vi "Main FPGA 8-axis.vi"() -> ()   [LabVIEW 2015]
uses:
  <vilib>/Motion/MotorControl/_s/nism.interpretControlRegister.stateTransition.ctl
  <vilib>/Platform/TimedLoop/XDataNode/timing_clust.ctl
  <vilib>/Platform/TimedLoop/XDataNode/nitl_modes.ctl
  <vilib>/Platform/TimedLoop/XDataNode/wakeup.ctl
  <vilib>/rvi/Emulation/niFpgaGetClockAttributes.vi
  <vilib>/rvi/Emulation/niFpgaSctlEmulationGetInTimedLoop.vi
  <vilib>/rvi/Emulation/niFpgaEmulationReportErrorSimple.vi
  Global FPGA 8-axis.vi
  <vilib>/Motion/MotorControl/_s/nism.interpretControlRegister.indexed.vi
  <vilib>/rvi/Emulation/niFpgaProcessEmulError.vi
  <vilib>/Motion/MotorControl/_s/nism.mdo.read.positionLoopSyncData.vi
  <vilib>/Motion/MotorControl/_s/nism.mdo.read.splineData.vi
  <vilib>/Motion/MotorControl/_s/nism.generateStatusRegister.indexed.vi
  <vilib>/rvi/eio/common/nirviEmuTemplateMethod_errors.vi
  <vilib>/rvi/Emulation/niFpgaCriticalErrorInLSC.vi
  <vilib>/Motion/MotorControl/_s/nism.splineInterpolation.fxp.3.index.vi
  <vilib>/Motion/MotorControl/_s/nism.mdo.handler.indexed.vi
  <vilib>/Motion/SoftMotion/Synchronization/nism.rioScan.generateSyncScan.vi
  <vilib>/eio/EIONode/EIONode.xnode
  <vilib>/Platform/TimedLoop/XDataNode/XDataNode.xnode
  <vilib>/Motion/MotorControl/NI_SoftMotion_MotorControlIP.lvlib
  <vilib>/Platform/TimedLoop/XDataNode/XDNodeRunTimeDep.lvlib
  <vilib>/Motion/SoftMotion/Synchronization/NI_SoftMotion_Synchronization.lvlib
panel:
  out "Interpolated Positions":fxp<+/-,64,32>[](array[numeric])
  out "Drive Enable":bool[](array[boolean])
  in  "Enable value":bool
  in  "Drive Enable override?":bool
  out "State":T1=enum."Start --> Initializing" caption="state transition"
  in  "Sync Value":bool
  in  "Sync Enable override?":bool
  in  "Invert direction?":bool
  out "Sync is Fault":bool
  out "Sync is Locked":bool
  in  "minimum pulse":u16=40
  # "Synchronization Loop"
  # "Control Status Loop"
  # "Notes: \n1. This VI provides the communication interface between the NI SoftMotion Engine and the LabVIEW FPGA Module. You must compile this VI for a specific FPGA target before use. After compiling, run the VI before running any of the Express VI examples. For information on moving this example to another FPGA target, refer to ni.com/info and enter info code fpgaex.\n\n2. Only use the Reset Axis button if you are unable to communicate with the axis by any other means. This button resets the device state machine and other VIs to a known state. After resetting the axis, switch the NI Scan Engine from Active Mode to Configuration Mode, then back to Active Mode, before attempting to enable the axis."
  # "(These two buttons \nare for testing\npurposes.)"
  # "(These two buttons \nare for testing\npurposes.)"
  # "Step/Direction Loop"
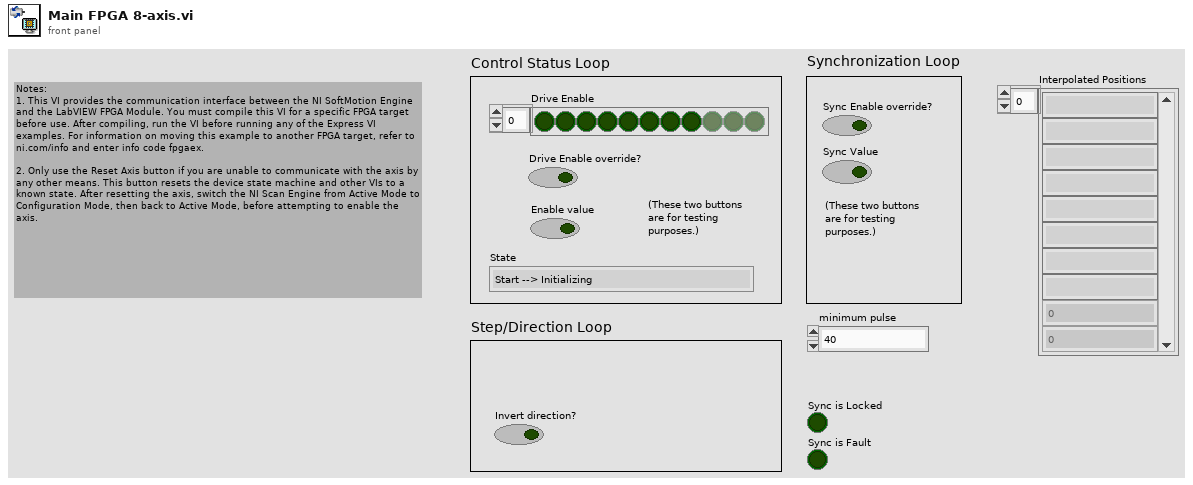
[diagram p1: front panel]
types:
  T1 = typedef "NI_SoftMotion_MotorControlIP.lvlib/nism.interpretControlRegister.stateTransition.ctl" = enum8{"Invalid", "Start --> Initializing", "Initializing --> Disabled", "Disabled --> Ready To Switch On", "Ready To Switch On --> Switched On", "Ready To Switch On --> Disable", "Switched On --> Operation Enable", "Switched On --> Ready To Switch On", "Switched On --> Disabled", "Operation Enable --> Switched On", "Operation Enable --> Ready To Switch On", "Operation Enable --> Disabled", "Fault --> Disabled", "Any --> Fault", "None"}
  T2 = typedef "NI_SoftMotion_MotorControlIP.lvlib/nism.mdo.splineData.ctl" = cluster{"spline type":T3, "traj per/spline per":u16, "spline per/traj per":fxp<+,32,0>}
  T3 = typedef "NI_SoftMotion_MotorControlIP.lvlib/nism.splineInterpolation.type.ctl" = u16
  T4 = typedef "NI_SoftMotion_Synchronization.lvlib/nism.softmotionScan.timerConfig.ctl" = cluster{"target period (clocks)":u16, "host period / target period":u16}
  T5 = typedef "NI_SoftMotion_Synchronization.lvlib/nism.softmotionScan.timerControl.ctl" = cluster{"sm scan":bool, "sm scan count":u32, "sm scan enabled":bool}
  T6 = typedef "XDNodeRunTimeDep.lvlib/timing_clust.ctl" = cluster{"Expected End [f-1]":u64, "Actual End [f-1]":u64, "Finished Late? [f-1]":bool, "Expected End [i-1]":u64, "Actual End [i-1]":u64, "Finished Late? [i-1]":bool, "Expected Start [i]":u64, "Actual Start [i]":u64, "Expected Start [f]":u64, "Actual Start [f]":u64, "Source Name":string, "Structure Name":string, "Period":i64, "Deadline":i64, "Offset":i64, "Start":i64, "Priority":i32, "Timeout":i32, "Mode":T7, "Wakeup Reason":T8, "Error":errorcluster, "Source Type":string, "Secondary Source Type":string, "Global End Time":u64, "Global Start Time":u64, "Frame Duration":u64, "Iteration Duration":u64, "Assigned CPU":i32, "I/O Scan Engine Mode":u32}
  T7 = typedef "XDNodeRunTimeDep.lvlib/nitl_modes.ctl" = enum32{"No Change", "Process missed periods, maintain original phase", "Discard missed periods, maintain original phase", "Process missed periods, ignore original phase", "Discard missed periods, ignore original phase"}
  T8 = typedef "XDNodeRunTimeDep.lvlib/wakeup.ctl" = enum32{"Normal", "Aborted", "Asynchronous wakeup", "Timing source error", "Timed loop error", "Timeout"}
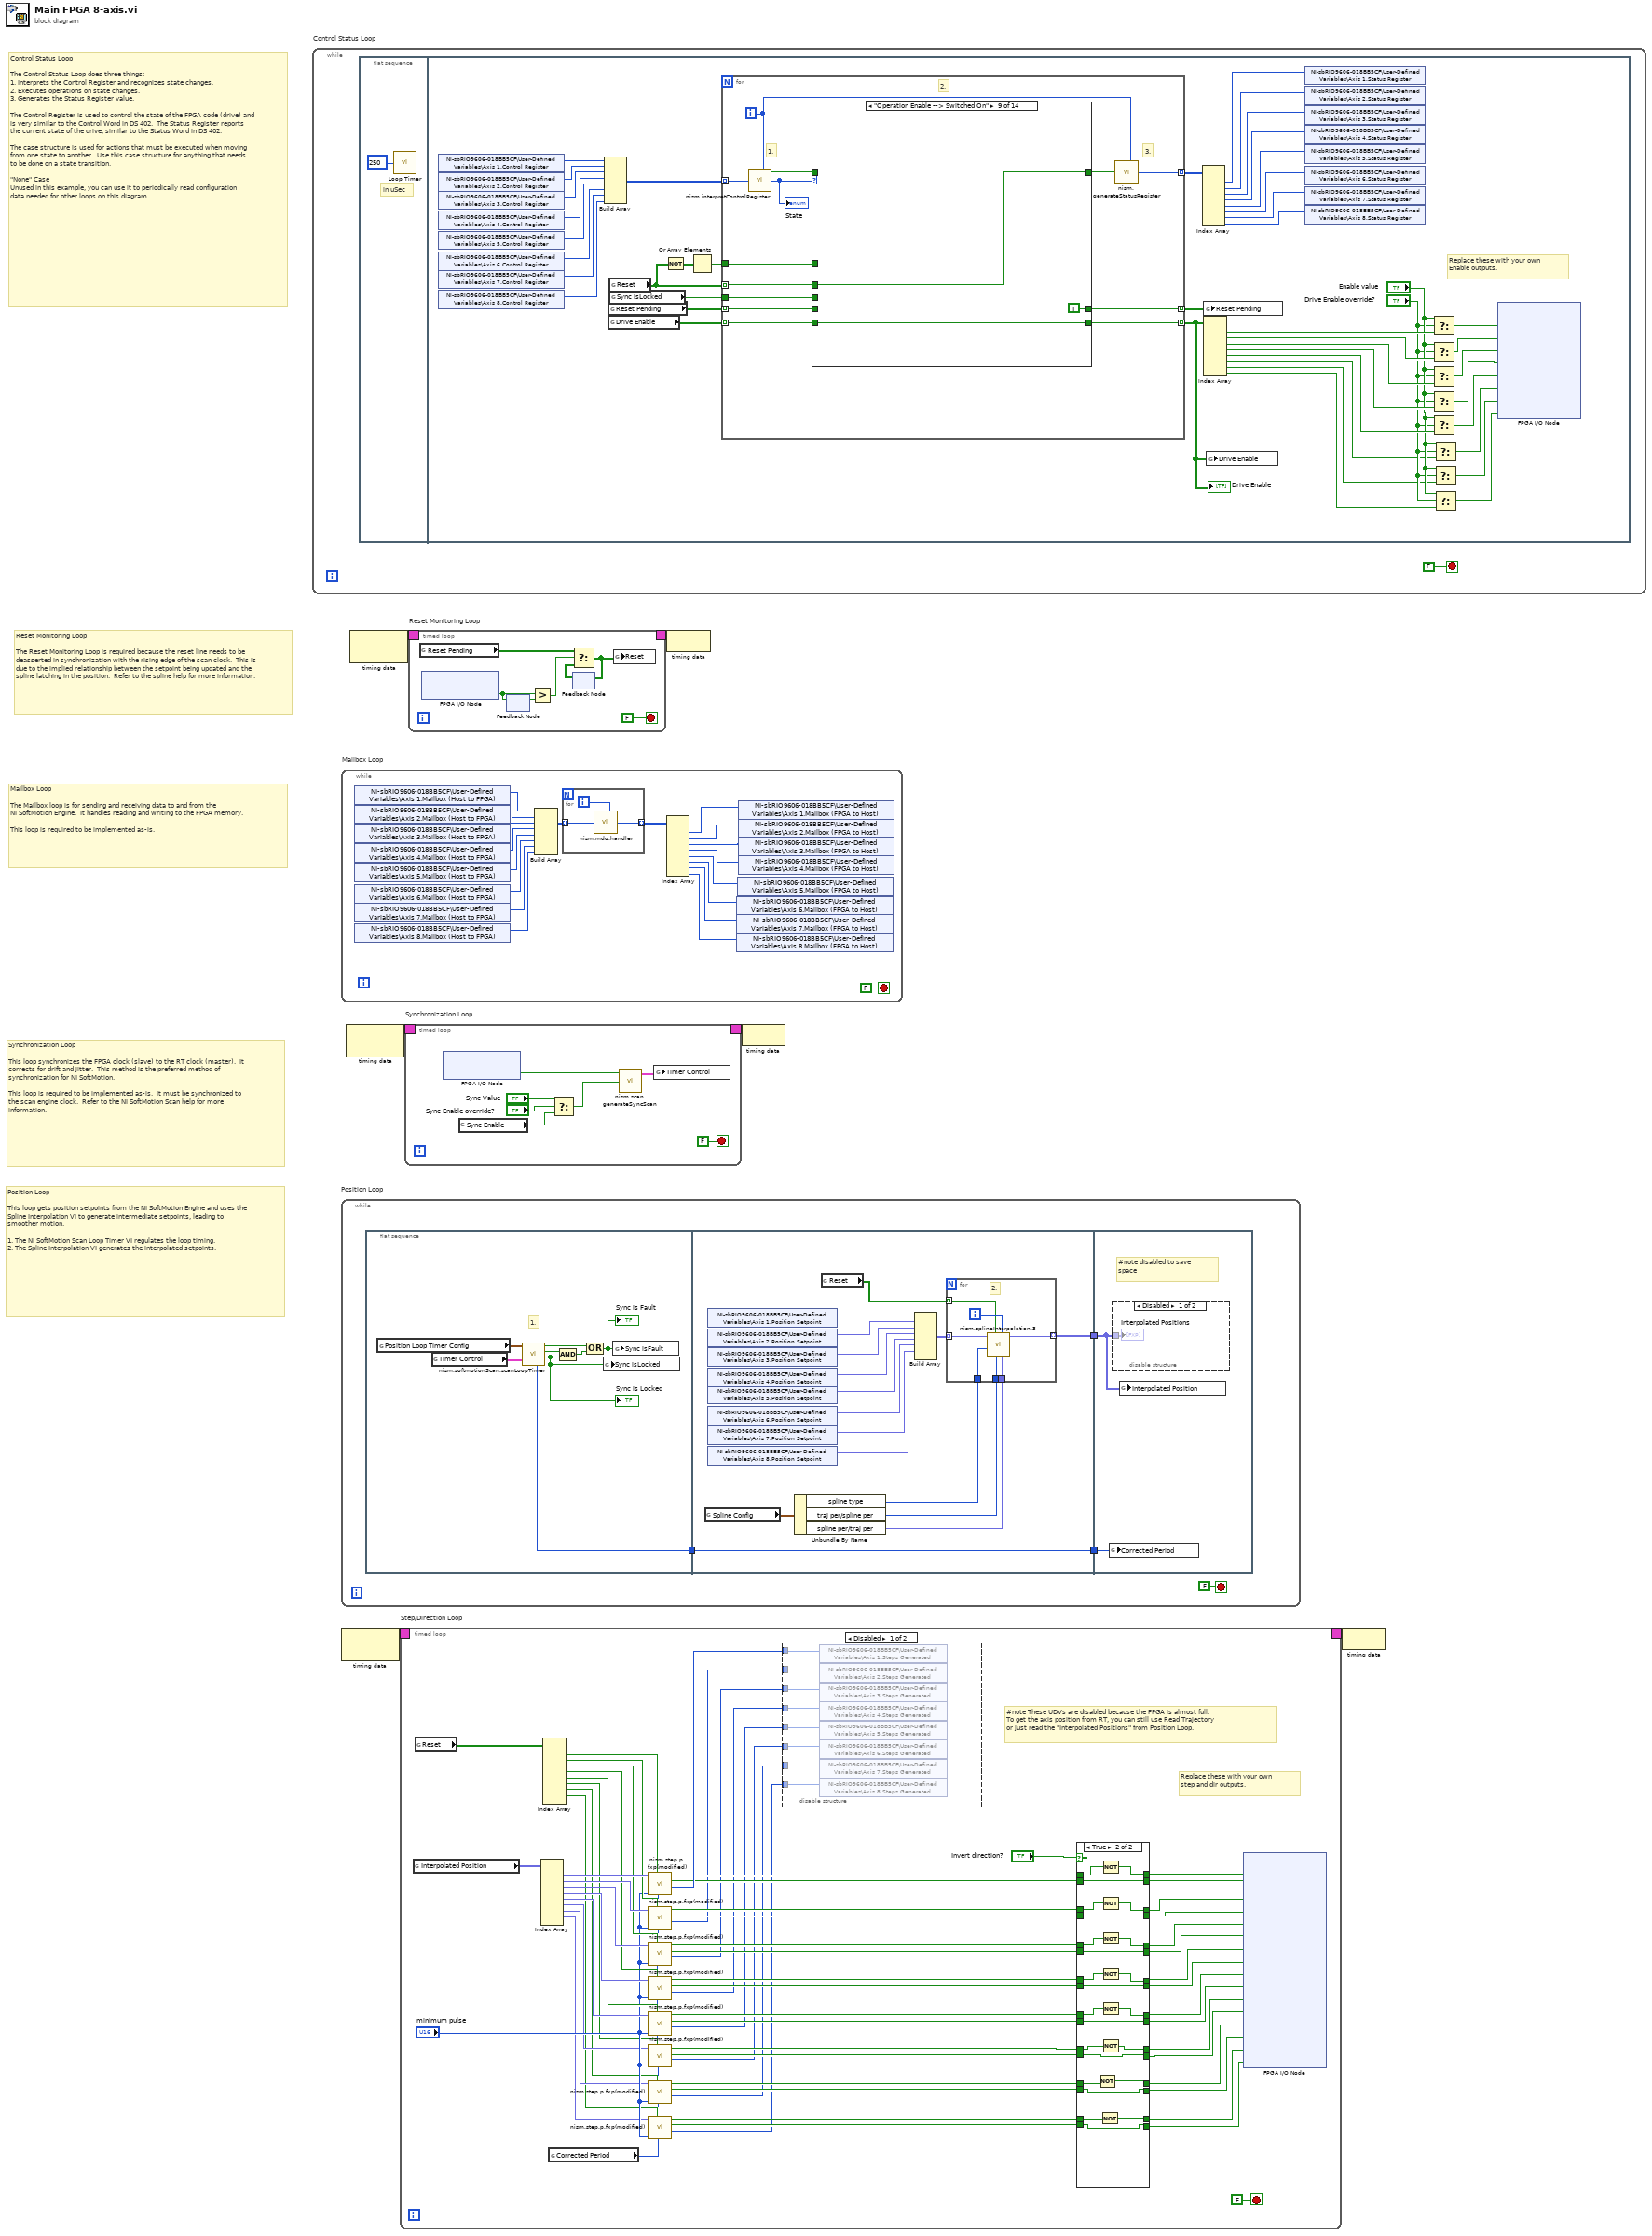
[diagram p0: block diagram]
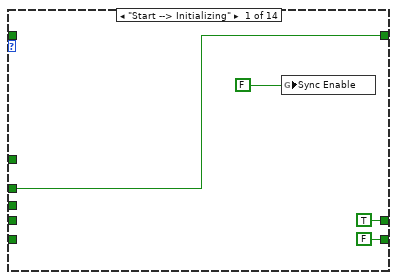
[diagram p5: hidden frame]
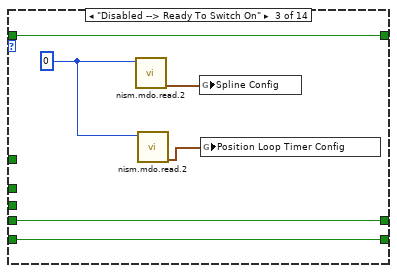
[diagram p7: hidden frame]
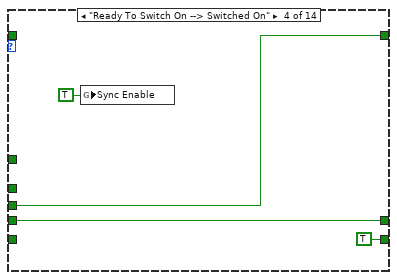
[diagram p8: hidden frame]
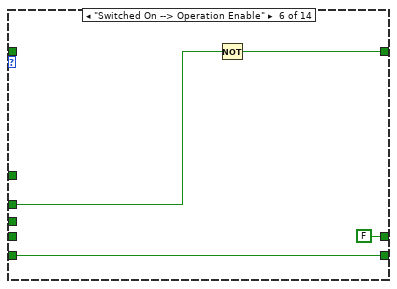
[diagram p10: hidden frame]
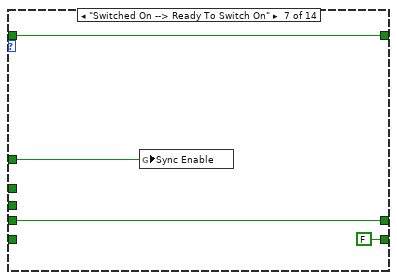
[diagram p11: hidden frame]
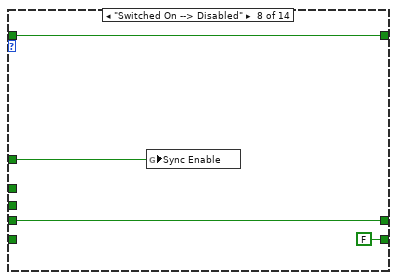
[diagram p12: hidden frame]
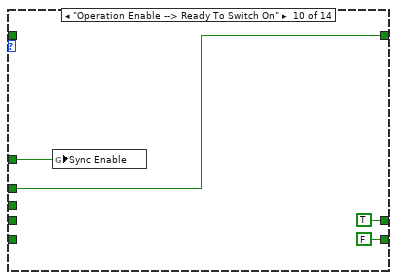
[diagram p13: hidden frame]
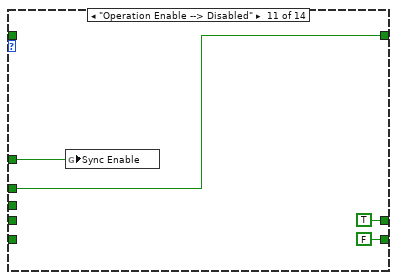
[diagram p14: hidden frame]
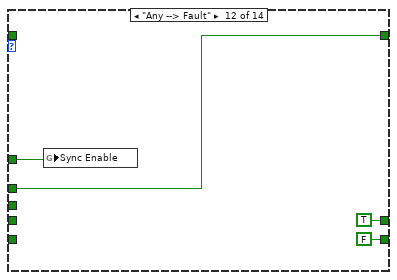
[diagram p15: hidden frame]
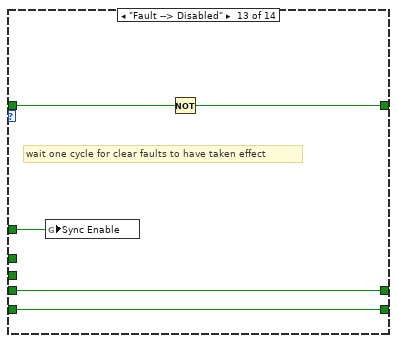
[diagram p16: hidden frame]
diagram:
  # "Position Loop\n\nThis loop gets position setpoints from the NI SoftMotion Engine and uses the Spline Interpolation VI to generate intermediate setpoints, leading to smoother motion.\n\n1. The NI SoftMotion Scan Loop Timer VI regulates the loop timing. \n2. The Spline Interpolation VI generates the interpolated setpoints."
  # "Synchronization Loop\n\nThis loop synchronizes the FPGA clock (slave) to the RT clock (master).  It corrects for drift and jitter.  This method is the preferred method of synchronization for NI SoftMotion.\n\nThis loop is required to be implemented as-is.  It must be synchronized to the scan engine clock.  Refer to the NI SoftMotion Scan help for more information."
  # "Mailbox Loop\n\nThe Mailbox loop is for sending and receiving data to and from the \nNI SoftMotion Engine.  It handles reading and writing to the FPGA memory.\n\nThis loop is required to be implemented as-is."
  # "Reset Monitoring Loop\n\nThe Reset Monitoring Loop is required because the reset line needs to be deasserted in synchronization with the rising edge of the scan clock.  This is due to the implied relationship between the setpoint being updated and the spline latching in the position.  Refer to the spline help for more information."
  # "Control Status Loop\n\nThe Control Status Loop does three things:\n1. Interprets the Control Register and recognizes state changes.\n2. Executes operations on state changes.\n3. Generates the Status Register value.\n\nThe Control Register is used to control the state of the FPGA code (drive) and is very similar to the Control Word in DS 402.  The Status Register reports the current state of the drive, similar to the Status Word in DS 402.\n\nThe case structure is used for actions that must be executed when moving from one state to another.  Use this case structure for anything that needs to be done on a state transition.\n\n\"None\" Case\nUnused in this example, you can use it to periodically read configuration data needed for other loops on this diagram."
  n1 = while "Control Status Loop" {
    stop <- FALSE stop-if-true
    n2 = flat-sequence {
      frame #0 {
        # "in uSec"
        n3 = call "Loop Timer"("Count(uSec)"=u32 250) -> ()  [unwired: 1 out]
      }
      frame #1 {
        # "Replace these with your own\nEnable outputs."
        n4 = shared-variable "NI-sbRIO9606-018BB5CF\\User-Defined Variables\\Axis 1.Control Register"() -> (w42:u32)  [unwired: 1 in, 1 out]
        n5 = shared-variable "NI-sbRIO9606-018BB5CF\\User-Defined Variables\\Axis 2.Control Register"() -> (w41:u32)  [unwired: 1 in, 1 out]
        n6 = shared-variable "NI-sbRIO9606-018BB5CF\\User-Defined Variables\\Axis 3.Control Register"() -> (w40:u32)  [unwired: 1 in, 1 out]
        n7 = shared-variable "NI-sbRIO9606-018BB5CF\\User-Defined Variables\\Axis 4.Control Register"() -> (w39:u32)  [unwired: 1 in, 1 out]
        n8 = shared-variable "NI-sbRIO9606-018BB5CF\\User-Defined Variables\\Axis 5.Control Register"() -> (w38:u32)  [unwired: 1 in, 1 out]
        n9 = shared-variable "NI-sbRIO9606-018BB5CF\\User-Defined Variables\\Axis 6.Control Register"() -> (w27:u32)  [unwired: 1 in, 1 out]
        n10 = shared-variable "NI-sbRIO9606-018BB5CF\\User-Defined Variables\\Axis 7.Control Register"() -> (w26:u32)  [unwired: 1 in, 1 out]
        n11 = shared-variable "NI-sbRIO9606-018BB5CF\\User-Defined Variables\\Axis 8.Control Register"() -> (w25:u32)  [unwired: 1 in, 1 out]
        n12 = Build Array(w42, w41, w40, w39, w38, w27, w26, w25) -> (w51:u32[])
        n13 = global read "Global FPGA 8-axis.vi" "Reset Pending"() -> (w46:bool[])
        n14 = global read "Global FPGA 8-axis.vi" "Drive Enable"() -> (w45:bool[])
        n15 = global read "Global FPGA 8-axis.vi" "Reset"() -> (w47:bool[])
        n16 = global read "Global FPGA 8-axis.vi" "Sync isLocked"() -> (w52:bool)
        n17 = Not(x=w47) -> (.not. x?=w49:bool[])
        n18 = Or Array Elements(Boolean array=w49) -> (logical OR=w48:bool)
        n19 = for {
          tunnel: w47 -> [w60] mode=indexing
          tunnel: w52 -> [w59]
          tunnel: w51 -> [w61] mode=indexing
          tunnel: [w58] -> w43 mode=indexing
          tunnel: [w57] -> w50 mode=indexing
          tunnel: [w56] -> w44 mode=indexing
          tunnel: w48 -> [w55]
          tunnel: w46 -> [w54] mode=indexing
          tunnel: w45 -> [w53] mode=indexing
          i -> [w62]
          # "3."
          # "2."
          # "1."
          n20 = call-poly <vilib>:"nism.interpretControlRegister.vi"("control register"=w61, "axis index"=w62) -> ("transition occurred"=w63:bool, "state transition"=w64:T1)  [unwired: 6 in]
          "State" <- w64
          n21 = case shown="\"Operation Enable --> Switched On\"" w64 {
            tunnel: w63 -> [_ w72 w78 _ w85 _ w93 w97 _ _ _ _ w117 _]
            tunnel: [w69 w72 w78 w80 w85 w89 w93 w97 w99 w102 w106 w110 w116 _] -> w65
            tunnel: w60 -> [w69 _ _ _ _ w88 _ _ w99 w102 w106 w110 _ _]
            tunnel: w59 -> [_ _ _ w80 _ _ _ _ _ _ _ _ _ _]
            tunnel: [TRUE ("Write.Reset Pending") w71 w74 w79 w84 FALSE ("Write.Reset Pending") w90 w94 TRUE ("Write.Reset Pending") TRUE ("Write.Reset Pending") TRUE ("Write.Reset Pending") TRUE ("Write.Reset Pending") w114 w119] -> w57
            tunnel: [FALSE ("Write.Drive Enable") w70 w73 TRUE ("Write.Drive Enable") w83 w86 FALSE ("Write.Drive Enable") FALSE ("Write.Drive Enable") w98 FALSE ("Write.Drive Enable") FALSE ("Write.Drive Enable") FALSE ("Write.Drive Enable") w113 w118] -> w56
            tunnel: w55 -> [_ _ _ _ _ _ w91 w95 _ w101 w105 w109 w115 _]
            tunnel: w54 -> [_ w71 w74 w79 w84 _ w90 w94 _ _ _ _ w114 w119]
            tunnel: w53 -> [_ w70 w73 _ w83 w86 _ _ w98 _ _ _ w113 w118]
            frame "Start --> Initializing" {
              n22 = global write "Global FPGA 8-axis.vi" "Sync Enable"(FALSE ("Sync Enable")) -> ()
            }
            frame "Initializing --> Disabled" {
            }
            frame "Disabled --> Ready To Switch On" {
              w76 = 0 ("axis index")
              n23 = call-poly <vilib>:"nism.mdo.read.2.vi"("axis index"=w76) -> ("spline"=w77:T2)  [unwired: 10 in]
              n24 = call-poly <vilib>:"nism.mdo.read.2.vi"("axis index"=w76) -> ("position loop sync"=w75:T4)  [unwired: 10 in]
              n25 = global write "Global FPGA 8-axis.vi" "Spline Config"(w77) -> ()
              n26 = global write "Global FPGA 8-axis.vi" "Position Loop Timer Config"(w75) -> ()
            }
            frame "Ready To Switch On --> Switched On" {
              n27 = global write "Global FPGA 8-axis.vi" "Sync Enable"(TRUE ("Sync Enable")) -> ()
            }
            frame "Ready To Switch On --> Disable" {
            }
            frame "Switched On --> Operation Enable" {
              n28 = Not(x=w88) -> (.not. x?=w89:bool)
            }
            frame "Switched On --> Ready To Switch On" {
              n29 = global write "Global FPGA 8-axis.vi" "Sync Enable"(w91) -> ()
            }
            frame "Switched On --> Disabled" {
              n30 = global write "Global FPGA 8-axis.vi" "Sync Enable"(w95) -> ()
            }
            frame "Operation Enable --> Switched On" {
            }
            frame "Operation Enable --> Ready To Switch On" {
              n31 = global write "Global FPGA 8-axis.vi" "Sync Enable"(w101) -> ()
            }
            frame "Operation Enable --> Disabled" {
              n32 = global write "Global FPGA 8-axis.vi" "Sync Enable"(w105) -> ()
            }
            frame "Any --> Fault" {
              n33 = global write "Global FPGA 8-axis.vi" "Sync Enable"(w109) -> ()
            }
            frame "Fault --> Disabled" {
              # "wait one cycle for clear faults to have taken effect"
              n34 = global write "Global FPGA 8-axis.vi" "Sync Enable"(w115) -> ()
              n35 = Not(x=w117) -> (.not. x?=w116:bool)
            }
            frame "None", Default {
            }
          }
          n36 = call-poly <vilib>:"nism.generateStatusRegister.vi"("transition success"=w65, "axis index"=w62) -> ("status register"=w58:u32)  [unwired: 7 in]
        }
        "Drive Enable" <- w44
        n37 = Index Array(array=w43) -> (element #1=w37:u32, element #2=w36:u32, element #3=w35:u32, element #4=w34:u32, element #5=w33:u32, element #6=w24:u32, element #7=w23:u32, element #8=w22:u32)  [unwired: 8 in]
        n38 = global write "Global FPGA 8-axis.vi" "Reset Pending"(w50) -> ()
        n39 = Index Array(array=w44) -> (element #1=w32:bool, element #2=w31:bool, element #3=w30:bool, element #4=w29:bool, element #5=w28:bool, element #6=w19:bool, element #7=w18:bool, element #8=w17:bool)  [unwired: 8 in]
        n40 = global write "Global FPGA 8-axis.vi" "Drive Enable"(w44) -> ()
        n41 = shared-variable "NI-sbRIO9606-018BB5CF\\User-Defined Variables\\Axis 1.Status Register"(w37) -> ()  [unwired: 1 in, 1 out]
        n42 = shared-variable "NI-sbRIO9606-018BB5CF\\User-Defined Variables\\Axis 2.Status Register"(w36) -> ()  [unwired: 1 in, 1 out]
        n43 = shared-variable "NI-sbRIO9606-018BB5CF\\User-Defined Variables\\Axis 3.Status Register"(w35) -> ()  [unwired: 1 in, 1 out]
        n44 = shared-variable "NI-sbRIO9606-018BB5CF\\User-Defined Variables\\Axis 4.Status Register"(w34) -> ()  [unwired: 1 in, 1 out]
        n45 = shared-variable "NI-sbRIO9606-018BB5CF\\User-Defined Variables\\Axis 5.Status Register"(w33) -> ()  [unwired: 1 in, 1 out]
        n46 = shared-variable "NI-sbRIO9606-018BB5CF\\User-Defined Variables\\Axis 6.Status Register"(w24) -> ()  [unwired: 1 in, 1 out]
        n47 = shared-variable "NI-sbRIO9606-018BB5CF\\User-Defined Variables\\Axis 7.Status Register"(w23) -> ()  [unwired: 1 in, 1 out]
        n48 = shared-variable "NI-sbRIO9606-018BB5CF\\User-Defined Variables\\Axis 8.Status Register"(w22) -> ()  [unwired: 1 in, 1 out]
        n49 = Select(t="Enable value", s="Drive Enable override?", f=w32) -> (s? t:f=w13:bool)
        n50 = Select(t="Enable value", s="Drive Enable override?", f=w31) -> (s? t:f=w12:bool)
        n51 = Select(t="Enable value", s="Drive Enable override?", f=w30) -> (s? t:f=w11:bool)
        n52 = Select(t="Enable value", s="Drive Enable override?", f=w29) -> (s? t:f=w10:bool)
        n53 = Select(t="Enable value", s="Drive Enable override?", f=w28) -> (s? t:f=w9:bool)
        n54 = Select(t="Enable value", s="Drive Enable override?", f=w19) -> (s? t:f=w16:bool)
        n55 = Select(t="Enable value", s="Drive Enable override?", f=w18) -> (s? t:f=w15:bool)
        n56 = Select(t="Enable value", s="Drive Enable override?", f=w17) -> (s? t:f=w14:bool)
        n57 = xnode "FPGA I/O Node"("RMC/DIO15"=w13, "RMC/DIO79"=w12, "RMC/DIO78"=w11, "RMC/DIO13"=w10, "RMC/DIO62"=w9, "RMC/DIO61"=w16, "RMC/DIO76"=w15, "RMC/DIO11"=w14) -> ()  [unwired: 8 in, 8 out]
      }
    }
  }
  n58 = while "Position Loop" {
    stop <- FALSE stop-if-true
    n59 = flat-sequence {
      tunnel: [w124] -> w120
      tunnel: [w141] -> w122
      tunnel: [w140] -> w121
      tunnel: w120 -> [w140]
      tunnel: w122 -> [w155]
      tunnel: w121 -> [w156]
      frame #0 {
        # "1."
        n60 = global read "Global FPGA 8-axis.vi" "Position Loop Timer Config"() -> (w126:T4)
        n61 = global read "Global FPGA 8-axis.vi" "Timer Control"() -> (w125:T5)
        n62 = call <vilib>:"nism.softmotionScan.scanLoopTimer.vi"("timer control"=w125, "timer config"=w126) -> ("scan running?"=w128:bool, "finished late?"=w130:bool, "fault occurred?"=w131:bool, "corrected period"=w124:u16)  [unwired: 5 in, 1 out]
        "Sync is Locked" <- w128
        n63 = Compound Arithmetic op=AND(w130, w128) -> (w129:bool)
        n64 = Compound Arithmetic op=OR(w131, w129) -> (w127:bool)
        "Sync is Fault" <- w127
        n65 = global write "Global FPGA 8-axis.vi" "Sync isLocked"(w128) -> ()
        n66 = global write "Global FPGA 8-axis.vi" "Sync isFault"(w127) -> ()
      }
      frame #1 {
        n67 = global read "Global FPGA 8-axis.vi" "Spline Config"() -> (w143:T2)
        n68 = shared-variable "NI-sbRIO9606-018BB5CF\\User-Defined Variables\\Axis 1.Position Setpoint"() -> (w139:fxp<+/-,64,32>)  [unwired: 1 in, 1 out]
        n69 = shared-variable "NI-sbRIO9606-018BB5CF\\User-Defined Variables\\Axis 2.Position Setpoint"() -> (w138:fxp<+/-,64,32>)  [unwired: 1 in, 1 out]
        n70 = shared-variable "NI-sbRIO9606-018BB5CF\\User-Defined Variables\\Axis 3.Position Setpoint"() -> (w137:fxp<+/-,64,32>)  [unwired: 1 in, 1 out]
        n71 = shared-variable "NI-sbRIO9606-018BB5CF\\User-Defined Variables\\Axis 4.Position Setpoint"() -> (w136:fxp<+/-,64,32>)  [unwired: 1 in, 1 out]
        n72 = shared-variable "NI-sbRIO9606-018BB5CF\\User-Defined Variables\\Axis 5.Position Setpoint"() -> (w135:fxp<+/-,64,32>)  [unwired: 1 in, 1 out]
        n73 = shared-variable "NI-sbRIO9606-018BB5CF\\User-Defined Variables\\Axis 6.Position Setpoint"() -> (w134:fxp<+/-,64,32>)  [unwired: 1 in, 1 out]
        n74 = shared-variable "NI-sbRIO9606-018BB5CF\\User-Defined Variables\\Axis 7.Position Setpoint"() -> (w133:fxp<+/-,64,32>)  [unwired: 1 in, 1 out]
        n75 = shared-variable "NI-sbRIO9606-018BB5CF\\User-Defined Variables\\Axis 8.Position Setpoint"() -> (w132:fxp<+/-,64,32>)  [unwired: 1 in, 1 out]
        n76 = Unbundle By Name(w143) -> ("spline type"=w147:T3, "traj per/spline per"=w146:u16, "spline per/traj per"=w145:fxp<+,32,0>)
        n77 = global read "Global FPGA 8-axis.vi" "Reset"() -> (w142:bool[])
        n78 = Build Array(w139, w138, w137, w136, w135, w134, w133, w132) -> (w144:fxp<+/-,64,32>[])
        n79 = for {
          tunnel: w147 -> [w154]
          tunnel: w146 -> [w153]
          tunnel: w145 -> [w152]
          tunnel: w142 -> [w149] mode=indexing
          tunnel: w144 -> [w151] mode=indexing
          tunnel: [w148] -> w141 mode=indexing
          i -> [w150]
          # "2."
          n80 = call-poly <vilib>:"nism.splineInterpolation.3.vi"("1 / calls per sample"=w152, "index"=w150, "calls per sample"=w153, "reset"=w149, "spline type"=w154, "x"=w151) -> ("xi"=w148:fxp<+/-,64,32>)  [unwired: 4 in, 1 out]
        }
      }
      frame #2 {
        # "#note disabled to save \nspace"
        n81 = global write "Global FPGA 8-axis.vi" "Corrected Period"(w156) -> ()
        n82 = disable-structure shown="Disabled" {
          disable-tunnel: w155 -> [w157 _]
          frame Disabled {
            "Interpolated Positions" <- w157
          }
          frame Enabled {
          }
        }
        n83 = global write "Global FPGA 8-axis.vi" "Interpolated Position"(w155) -> ()
      }
    }
  }
  n84 = node-c288() -> (w6:T6)  [unwired: 1 in]
  n85 = while "Mailbox Loop" {
    stop <- FALSE stop-if-true
    n86 = shared-variable "NI-sbRIO9606-018BB5CF\\User-Defined Variables\\Axis 1.Mailbox (Host to FPGA)"() -> (w173:u64)  [unwired: 1 in, 1 out]
    n87 = shared-variable "NI-sbRIO9606-018BB5CF\\User-Defined Variables\\Axis 2.Mailbox (Host to FPGA)"() -> (w172:u64)  [unwired: 1 in, 1 out]
    n88 = shared-variable "NI-sbRIO9606-018BB5CF\\User-Defined Variables\\Axis 3.Mailbox (Host to FPGA)"() -> (w171:u64)  [unwired: 1 in, 1 out]
    n89 = shared-variable "NI-sbRIO9606-018BB5CF\\User-Defined Variables\\Axis 4.Mailbox (Host to FPGA)"() -> (w170:u64)  [unwired: 1 in, 1 out]
    n90 = shared-variable "NI-sbRIO9606-018BB5CF\\User-Defined Variables\\Axis 5.Mailbox (Host to FPGA)"() -> (w169:u64)  [unwired: 1 in, 1 out]
    n91 = shared-variable "NI-sbRIO9606-018BB5CF\\User-Defined Variables\\Axis 6.Mailbox (Host to FPGA)"() -> (w163:u64)  [unwired: 1 in, 1 out]
    n92 = shared-variable "NI-sbRIO9606-018BB5CF\\User-Defined Variables\\Axis 7.Mailbox (Host to FPGA)"() -> (w162:u64)  [unwired: 1 in, 1 out]
    n93 = shared-variable "NI-sbRIO9606-018BB5CF\\User-Defined Variables\\Axis 8.Mailbox (Host to FPGA)"() -> (w161:u64)  [unwired: 1 in, 1 out]
    n94 = Build Array(w173, w172, w171, w170, w169, w163, w162, w161) -> (w175:u64[])
    n95 = for {
      tunnel: w175 -> [w179] mode=indexing
      tunnel: [w178] -> w174 mode=indexing
      i -> [w177]
      n96 = call-poly <vilib>:"nism.mdo.handler.vi"("mbox (host to fpga)"=w179, "axis index"=w177) -> ("mbox (fpga to host)"=w178:u64)  [unwired: 7 in]
    }
    n97 = Index Array(array=w174) -> (element #1=w168:u64, element #2=w167:u64, element #3=w166:u64, element #4=w165:u64, element #5=w164:u64, element #6=w160:u64, element #7=w159:u64, element #8=w158:u64)  [unwired: 8 in]
    n98 = shared-variable "NI-sbRIO9606-018BB5CF\\User-Defined Variables\\Axis 6.Mailbox (FPGA to Host)"(w160) -> ()  [unwired: 1 in, 1 out]
    n99 = shared-variable "NI-sbRIO9606-018BB5CF\\User-Defined Variables\\Axis 7.Mailbox (FPGA to Host)"(w159) -> ()  [unwired: 1 in, 1 out]
    n100 = shared-variable "NI-sbRIO9606-018BB5CF\\User-Defined Variables\\Axis 8.Mailbox (FPGA to Host)"(w158) -> ()  [unwired: 1 in, 1 out]
    n101 = shared-variable "NI-sbRIO9606-018BB5CF\\User-Defined Variables\\Axis 5.Mailbox (FPGA to Host)"(w164) -> ()  [unwired: 1 in, 1 out]
    n102 = shared-variable "NI-sbRIO9606-018BB5CF\\User-Defined Variables\\Axis 1.Mailbox (FPGA to Host)"(w168) -> ()  [unwired: 1 in, 1 out]
    n103 = shared-variable "NI-sbRIO9606-018BB5CF\\User-Defined Variables\\Axis 2.Mailbox (FPGA to Host)"(w167) -> ()  [unwired: 1 in, 1 out]
    n104 = shared-variable "NI-sbRIO9606-018BB5CF\\User-Defined Variables\\Axis 3.Mailbox (FPGA to Host)"(w166) -> ()  [unwired: 1 in, 1 out]
    n105 = shared-variable "NI-sbRIO9606-018BB5CF\\User-Defined Variables\\Axis 4.Mailbox (FPGA to Host)"(w165) -> ()  [unwired: 1 in, 1 out]
  }
  n106 = node-c288() -> (w4:T6)  [unwired: 1 in]
  n107 = node-c288() -> (w2:T6)  [unwired: 1 in]
  n108 = timed-loop "Step/Direction Loop" {
    timing: w6 -> [_]
    timing-out: [_] -> w5
    stop <- FALSE stop-if-true
    # "#note These UDVs are disabled because the FPGA is almost full.\nTo get the axis position from RT, you can still use Read Trajectory\nor just read the \"Interpolated Positions\" from Position Loop."
    # "Replace these with your own\nstep and dir outputs."
    n109 = global read "Global FPGA 8-axis.vi" "Interpolated Position"() -> (w240:fxp<+/-,64,32>[])
    n110 = global read "Global FPGA 8-axis.vi" "Reset"() -> (w234:bool[])
    n111 = Index Array(array=w240) -> (element #1=w239:fxp<+/-,64,32>, element #2=w238:fxp<+/-,64,32>, element #3=w237:fxp<+/-,64,32>, element #4=w236:fxp<+/-,64,32>, element #5=w235:fxp<+/-,64,32>, element #6=w202:fxp<+/-,64,32>, element #7=w201:fxp<+/-,64,32>, element #8=w200:fxp<+/-,64,32>)  [unwired: 9 in, 1 out]
    n112 = Index Array(array=w234) -> (element #1=w233:bool, element #2=w232:bool, element #3=w231:bool, element #4=w230:bool, element #5=w229:bool, element #6=w199:bool, element #7=w198:bool, element #8=w197:bool)  [unwired: 9 in, 1 out]
    n113 = global read "Global FPGA 8-axis.vi" "Corrected Period"() -> (w190:u16)
    n114 = call "nism.step.p.fxp(modified).vi"("calls per sample"=w190, "reset"=w233, "minimum pulse"="minimum pulse", "position setpoint"=w239) -> ("steps generated"=w228:i32, "step"=w226:bool, "direction"=w227:bool)  [unwired: 4 in, 1 out]
    n115 = call "nism.step.p.fxp(modified).vi"("calls per sample"=w190, "reset"=w232, "minimum pulse"="minimum pulse", "position setpoint"=w238) -> ("steps generated"=w217:i32, "step"=w224:bool, "direction"=w225:bool)  [unwired: 4 in, 1 out]
    n116 = call "nism.step.p.fxp(modified).vi"("calls per sample"=w190, "reset"=w231, "minimum pulse"="minimum pulse", "position setpoint"=w237) -> ("steps generated"=w216:i32, "step"=w222:bool, "direction"=w223:bool)  [unwired: 4 in, 1 out]
    n117 = call "nism.step.p.fxp(modified).vi"("calls per sample"=w190, "reset"=w230, "minimum pulse"="minimum pulse", "position setpoint"=w236) -> ("steps generated"=w215:i32, "step"=w220:bool, "direction"=w221:bool)  [unwired: 4 in, 1 out]
    n118 = call "nism.step.p.fxp(modified).vi"("calls per sample"=w190, "reset"=w229, "minimum pulse"="minimum pulse", "position setpoint"=w235) -> ("steps generated"=w214:i32, "step"=w218:bool, "direction"=w219:bool)  [unwired: 4 in, 1 out]
    n119 = call "nism.step.p.fxp(modified).vi"("calls per sample"=w190, "reset"=w199, "minimum pulse"="minimum pulse", "position setpoint"=w202) -> ("steps generated"=w205:i32, "step"=w211:bool, "direction"=w212:bool)  [unwired: 4 in, 1 out]
    n120 = call "nism.step.p.fxp(modified).vi"("calls per sample"=w190, "reset"=w198, "minimum pulse"="minimum pulse", "position setpoint"=w201) -> ("steps generated"=w204:i32, "step"=w209:bool, "direction"=w210:bool)  [unwired: 4 in, 1 out]
    n121 = call "nism.step.p.fxp(modified).vi"("calls per sample"=w190, "reset"=w197, "minimum pulse"="minimum pulse", "position setpoint"=w200) -> ("steps generated"=w203:i32, "step"=w207:bool, "direction"=w208:bool)  [unwired: 4 in, 1 out]
    n122 = disable-structure shown="Disabled" {
      disable-tunnel: w228 -> [w249 _]
      disable-tunnel: w217 -> [w248 _]
      disable-tunnel: w216 -> [w247 _]
      disable-tunnel: w215 -> [w246 _]
      disable-tunnel: w214 -> [w245 _]
      disable-tunnel: w205 -> [w244 _]
      disable-tunnel: w204 -> [w243 _]
      disable-tunnel: w203 -> [w242 _]
      frame Disabled {
        n123 = shared-variable "NI-sbRIO9606-018BB5CF\\User-Defined Variables\\Axis 1.Steps Generated"(w249) -> ()  [unwired: 1 in, 1 out]
        n124 = shared-variable "NI-sbRIO9606-018BB5CF\\User-Defined Variables\\Axis 2.Steps Generated"(w248) -> ()  [unwired: 1 in, 1 out]
        n125 = shared-variable "NI-sbRIO9606-018BB5CF\\User-Defined Variables\\Axis 3.Steps Generated"(w247) -> ()  [unwired: 1 in, 1 out]
        n126 = shared-variable "NI-sbRIO9606-018BB5CF\\User-Defined Variables\\Axis 4.Steps Generated"(w246) -> ()  [unwired: 1 in, 1 out]
        n127 = shared-variable "NI-sbRIO9606-018BB5CF\\User-Defined Variables\\Axis 5.Steps Generated"(w245) -> ()  [unwired: 1 in, 1 out]
        n128 = shared-variable "NI-sbRIO9606-018BB5CF\\User-Defined Variables\\Axis 6.Steps Generated"(w244) -> ()  [unwired: 1 in, 1 out]
        n129 = shared-variable "NI-sbRIO9606-018BB5CF\\User-Defined Variables\\Axis 7.Steps Generated"(w243) -> ()  [unwired: 1 in, 1 out]
        n130 = shared-variable "NI-sbRIO9606-018BB5CF\\User-Defined Variables\\Axis 8.Steps Generated"(w242) -> ()  [unwired: 1 in, 1 out]
      }
      frame Enabled {
      }
    }
    n131 = case shown="True" "Invert direction?" {
      tunnel: w227 -> [w265 w289]
      tunnel: [w265 w288] -> w189
      tunnel: w225 -> [w263 w287]
      tunnel: [w263 w286] -> w187
      tunnel: w223 -> [w261 w285]
      tunnel: [w261 w284] -> w185
      tunnel: w221 -> [w259 w283]
      tunnel: [w259 w282] -> w183
      tunnel: w219 -> [w257 w281]
      tunnel: [w257 w280] -> w181
      tunnel: w226 -> [w264 w279]
      tunnel: [w264 w279] -> w188
      tunnel: w224 -> [w262 w278]
      tunnel: [w262 w278] -> w186
      tunnel: w222 -> [w260 w277]
      tunnel: [w260 w277] -> w184
      tunnel: w220 -> [w258 w276]
      tunnel: [w258 w276] -> w182
      tunnel: w218 -> [w256 w275]
      tunnel: [w256 w275] -> w180
      tunnel: w212 -> [w255 w274]
      tunnel: w211 -> [w254 w267]
      tunnel: w210 -> [w253 w273]
      tunnel: w209 -> [w252 w269]
      tunnel: w208 -> [w251 w272]
      tunnel: w207 -> [w250 w270]
      tunnel: [w255 w266] -> w196
      tunnel: [w254 w267] -> w195
      tunnel: [w253 w268] -> w194
      tunnel: [w252 w269] -> w193
      tunnel: [w251 w271] -> w192
      tunnel: [w250 w270] -> w191
      frame False {
      }
      frame True {
        n132 = Not(x=w273) -> (.not. x?=w268:bool)
        n133 = Not(x=w272) -> (.not. x?=w271:bool)
        n134 = Not(x=w289) -> (.not. x?=w288:bool)
        n135 = Not(x=w287) -> (.not. x?=w286:bool)
        n136 = Not(x=w285) -> (.not. x?=w284:bool)
        n137 = Not(x=w283) -> (.not. x?=w282:bool)
        n138 = Not(x=w281) -> (.not. x?=w280:bool)
        n139 = Not(x=w274) -> (.not. x?=w266:bool)
      }
    }
    n140 = xnode "FPGA I/O Node"("RMC/DIO46"=w189, "RMC/DIO47"=w188, "RMC/DIO14"=w187, "RMC/DIO63"=w186, "RMC/DIO95"=w185, "RMC/DIO31"=w184, "RMC/DIO30"=w183, "RMC/DIO45"=w182, "RMC/DIO77"=w181, "RMC/DIO44"=w180, "RMC/DIO12"=w196, "RMC/DIO94"=w195, "RMC/DIO93"=w194, "RMC/DIO29"=w193, "RMC/DIO28"=w192, "RMC/DIO43"=w191) -> ()  [unwired: 16 in, 16 out]
  }
  n141 = timed-loop "Synchronization Loop" {
    timing: w4 -> [_]
    timing-out: [_] -> w3
    stop <- FALSE stop-if-true
    n142 = xnode "FPGA I/O Node"() -> ("Scan Clock"=w296:bool)  [unwired: 1 in, 1 out]
    n143 = global read "Global FPGA 8-axis.vi" "Sync Enable"() -> (w295:bool)
    n144 = Select(t="Sync Value", s="Sync Enable override?", f=w295) -> (s? t:f=w292:bool)
    n145 = call-poly <vilib>:"nism.scan.generateSyncScan.vi"("scan enable?"=w292, "scan clock"=w296) -> ("timer control"=w297:T5)  [unwired: 3 in]
    n146 = global write "Global FPGA 8-axis.vi" "Timer Control"(w297) -> ()
  }
  n147 = timed-loop "Reset Monitoring Loop" {
    timing: w2 -> [_]
    timing-out: [_] -> w1
    stop <- FALSE stop-if-true
    n148 = global read "Global FPGA 8-axis.vi" "Reset Pending"() -> (w303:bool[])
    n149 = xnode "FPGA I/O Node"() -> ("Scan Clock"=w302:bool)  [unwired: 1 in, 1 out]
    n150 = feedback-in #1(w302) -> ()
    n151 = feedback #1() -> (w301:bool)  [unwired: 1 in]
    n152 = Greater?(x=w302, y=w301) -> (0:w307:bool)
    n153 = feedback #2() -> (w306:bool[])  [unwired: 1 in]
    n154 = Select(t=w303, s=w307, f=w306) -> (s? t:f=w304:bool[])
    n155 = feedback-in #2(w304) -> ()
    n156 = global write "Global FPGA 8-axis.vi" "Reset"(w304) -> ()
  }
  n157 = node-c288(w1) -> ()
  n158 = node-c288(w3) -> ()
  n159 = node-c288(w5) -> ()
